vi "PTSequencer.setup stop conditions.vi"(0 "stop conditions in":T1[](array[typedef]), 3 "Use stop conditions in":bool, 5 "error in (no error)":errorcluster, 6 "read only":bool) -> (14 "stop conditions out":T1[](array[typedef]), 16 "changed":bool, 17 "Use stop conditions out":bool, 19 "error out":errorcluster)   [LabVIEW 2014, in "PTSequencer.lvlib"]
uses:
  PTSequencer.lvlib
  _typedefs/X DIM conditions/X DIM conditions.xctl
  PTSequencer.DIM service condition.ctl
  CS_Core/CSSystem/CoreDefs/CoreDefs.rawDataType.ctl
  _common/PTUtils/PTUtils.lvlib
  CS_Core/CSSystem/CSSystemLib/CSSystemLib.lvlib
panel:
  in  "Cancel":bool
  in  "Ok":bool
  in  "Use stop conditions":bool
  in  "DIM Services":T3(xcontrol) caption="Stop conditions"
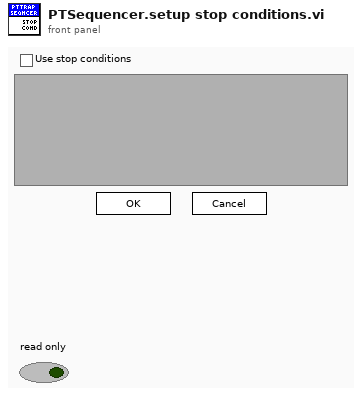
[diagram p1: front panel]
types:
  T1 = typedef "PTSequencer.lvlib/PTSequencer.DIM service condition.ctl" = cluster{"DIM service":string, "descr":string, "nomValue":T2, "actValue":T2, "matched":bool, "DIM Status":cluster{"no link":bool, "quality":i32, "Time Stamp":timestamp}}
  T2 = typedef "CoreDefs.rawDataType.ctl" = i8[]
  T3 = cluster{"DIM Services":string[], "data decsriptors":string[], "stop conditions":T1[]}
  T4 = enum8{"Enabled", "Disabled", "Disabled and Grayed Out"}
  T5 = cluster{"services":string[], "descriptors":string[], "Value":T1[]}
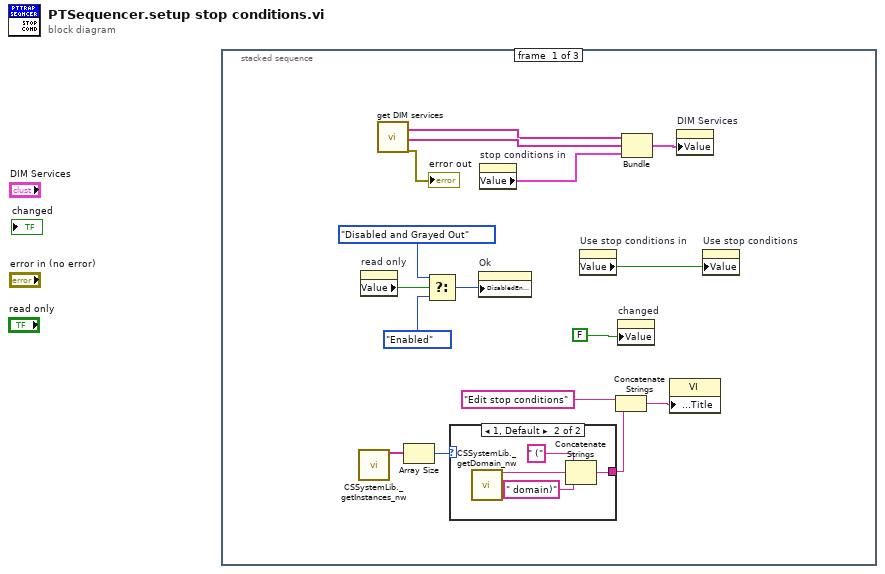
[diagram p0: block diagram]
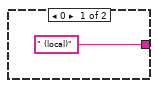
[diagram p2: hidden frame]
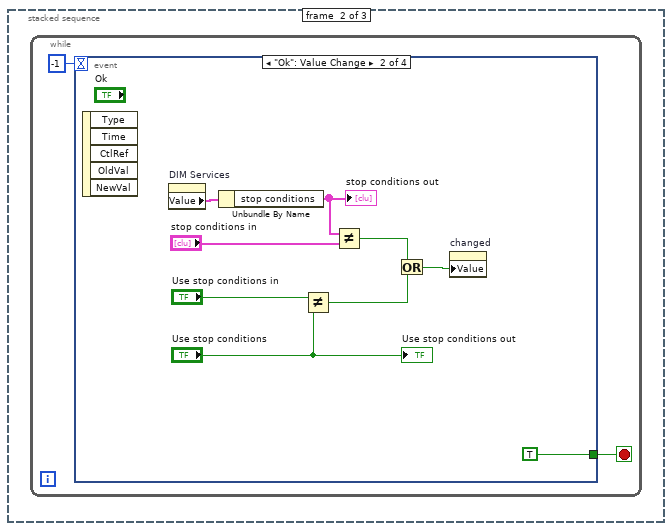
[diagram p3: hidden frame]
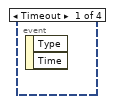
[diagram p4: hidden frame]
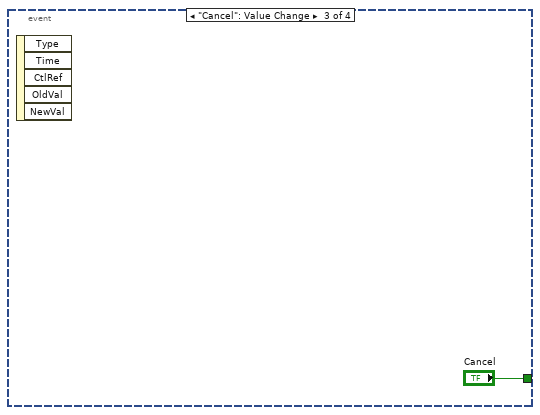
[diagram p5: hidden frame]
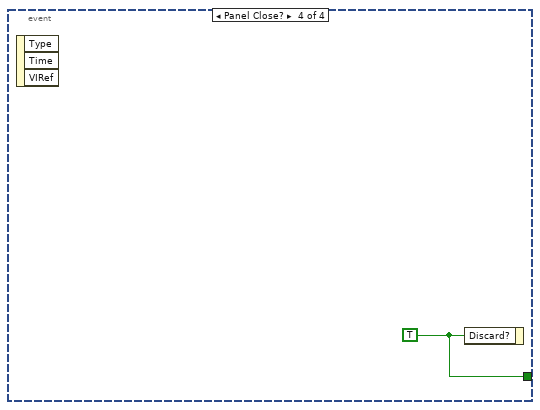
[diagram p6: hidden frame]
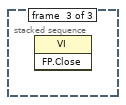
[diagram p7: hidden frame]
diagram:
  n1 = stacked-sequence {
    frame #0 {
      n2 = call "CSSystemLib._getInstances_nw.vi"() -> ("i list"=w8:string[])  [unwired: 18 in, 1 out]
      n3 = property on="read only" class="Bool (strict)"() -> ("Value"=w4:bool)  [unwired: 2 in, 2 out]
      n4 = call "get DIM services.vi"() -> ("services"=w13:string[], "descriptors"=w16:string[], "error out"=→"error out":errorcluster)  [unwired: 17 in]
      n5 = Array Size(array=w8) -> (size(s)=w9:i32)
      n6 = Select(t=T4."Disabled and Grayed Out" ("Disabled"), s=w4, f=T4."Enabled" ("Disabled")) -> (s? t:f=w1:T4)
      n7 = case shown="1, Default" w9 {
        tunnel: [" (local)" w18] -> w6
        frame 0 {
        }
        frame 1, Default {
          n8 = call "CSSystemLib._getDomain_nw.vi"() -> ("CSDomain"=w20:string)  [unwired: 18 in, 1 out]
          n9 = Concatenate Strings(" (", w20, " domain)") -> (w18:string)
        }
      }
      n10 = property on="Ok" class="Bool"("DisabledEnum"=w1) -> ()  [unwired: 2 in, 2 out]
      n11 = property on="stop conditions in" class="Arr (strict)"() -> ("Value"=w15:T1[])  [unwired: 2 in, 2 out]
      n12 = property on="Use stop conditions in" class="Bool (strict)"() -> ("Value"=w10:bool)  [unwired: 2 in, 2 out]
      n13 = Concatenate Strings("Edit stop conditions", w6) -> (w5:string)
      n14 = property on="changed" class="Bool (strict)"("Value"=FALSE ("changed")) -> ()  [unwired: 2 in, 2 out]
      n15 = Bundle("services"=w13, "descriptors"=w16, "Value"=w15) -> (w14:T5)  [unwired: 1 in]
      n16 = property class="VI"("Front Panel Window:Title"=w5) -> ()  [unwired: 2 in, 2 out]
      n17 = property on="DIM Services" class="X DIM conditions (strict)"("Value"=w14) -> ()  [unwired: 2 in, 2 out]
      n18 = property on="Use stop conditions" class="Bool (strict)"("Value"=w10) -> ()  [unwired: 2 in, 2 out]
    }
    frame #1 {
      n19 = while {
        stop <- w23 stop-if-true
        n20 = event shown="[1] \"Ok\": Value Change" {
          selector: _ -> [_ _ _ _]
          dyn-events: _ -> [_ _ _ _]
          timeout: -1 -> [_ _ _ _]
          tunnel: [_ TRUE "Cancel" w34] -> w23
          event Timeout {
            n21 = event-data() -> ()  [unwired: 1 in, 2 out]
          }
          event "Ok": Value Change {
            n22 = event-data() -> ()  [unwired: 1 in, 5 out]
            n23 = property on="DIM Services" class="X DIM conditions (strict)"() -> ("Value"=w32:T3)  [unwired: 2 in, 2 out]
            n24 = Unbundle By Name(w32) -> ("stop conditions"=w31:T1[])
            "stop conditions out" <- w31
            n25 = Not Equal?(x="Use stop conditions in", y="Use stop conditions") -> (x != y?=w28:bool)
            n26 = Not Equal?(x=w31, y="stop conditions in") -> (x != y?=w29:bool)
            n27 = Or(x=w29, y=w28) -> (x .or. y?=w27:bool)
            n28 = property on="changed" class="Bool (strict)"("Value"=w27) -> ()  [unwired: 2 in, 2 out]
            "Use stop conditions out" <- "Use stop conditions"
          }
          event "Cancel": Value Change {
            n29 = event-data() -> ()  [unwired: 1 in, 5 out]
          }
          event Panel Close? {
            w34 = TRUE
            n30 = event-data() -> ()  [unwired: 1 in, 3 out]
            n31 = event-data("Discard?"=w34) -> ()  [unwired: 1 in, 1 out]
          }
        }
      }
    }
    frame #2 {
      n32 = invoke class="VI" method="FP.Close"() -> ()  [unwired: 3 in, 3 out]
    }
  }
